vi "Read Multi Numeric as SGL.vi"(8 "error in (no error)":errorcluster, 9 "Type":sgl[](array[numeric]), 10 "Tag":string[](array[string]), 11 "Var Bus in":refnum<class "Omni_Bus.lvclass">) -> (0 "error out":errorcluster, 2 "Array":sgl[](array[numeric]), 3 "Var Bus out":refnum<class "Omni_Bus.lvclass">)   [LabVIEW 2021, in "Omni_Bus.lvclass"]
uses:
  Omni_Bus.lvclass
  <vilib>/TSA/Abstract Data Classes/Abs_Types/Numeric/Abs_Numeric.lvclass
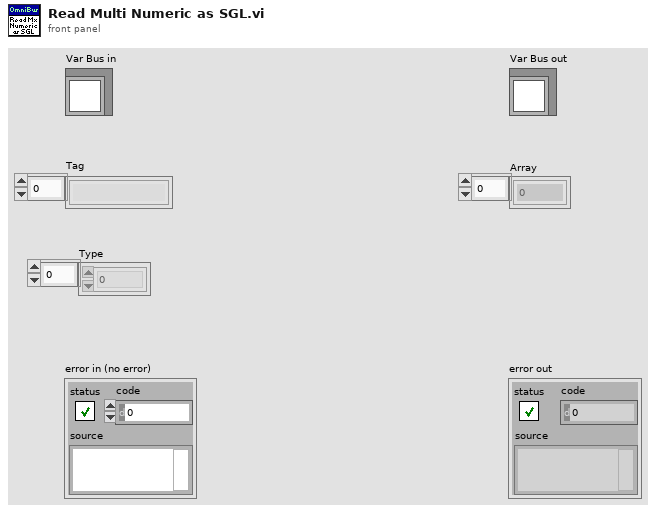
[diagram p1: front panel]
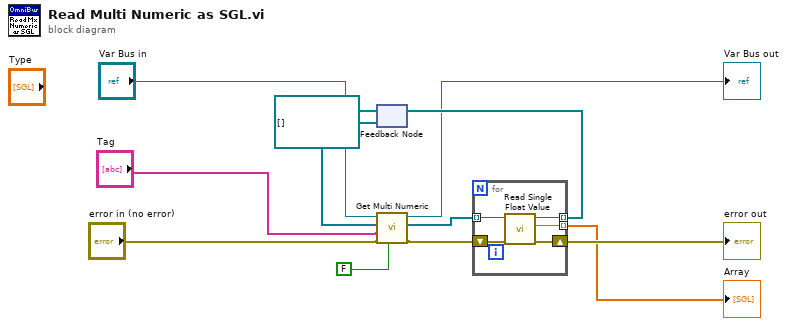
[diagram p0: block diagram]
diagram:
  n1 = feedback #1(refnum<class "Abs_Numeric.lvclass">[] []) -> (w5:refnum<class "Abs_Numeric.lvclass">[])
  n2 = call-dynamic "Get Multi Numeric.vi"("Write?"=FALSE, "error in (no error)"="error in (no error)", "Tag"="Tag", "Value Type"=w5, "Var Bus in"="Var Bus in") -> ("error out"=w9:errorcluster, "Value Out"=w8:refnum<class "Abs_Numeric.lvclass">[], "Var Bus out"=→"Var Bus out":refnum<class "Omni_Bus.lvclass">)  [unwired: 3 in, 1 out]
  n3 = for {
    tunnel: [w16] -> w11 mode=indexing
    tunnel: [w15] -> w10 mode=indexing
    tunnel: w8 -> [w13] mode=indexing
    shift-right: [w17] -> w12
    shift-left: w9 -> [w14]
    n4 = call-dynamic "Read Single Float Value.vi"("error in (no error)"=w14, "Numeric in"=w13) -> ("error out"=w17:errorcluster, "Float"=w16:sgl, "Numeric out"=w15:refnum<class "Abs_Numeric.lvclass">)  [unwired: 7 in]
  }
  "error out" <- w12
  "Array" <- w11
  n5 = feedback-in #1(w10) -> ()
